vi "QueuedMessageHandler 1.vi"   [LabVIEW 2012]
doc: "Use this template to build a queued message handler design pattern.\nNote: This template does not contain the most recent programming guidelines recommended by National Instruments. For a complete, project-based implementation of the Queued Message Handler pattern, use the Create Project dialog box instead of this template."
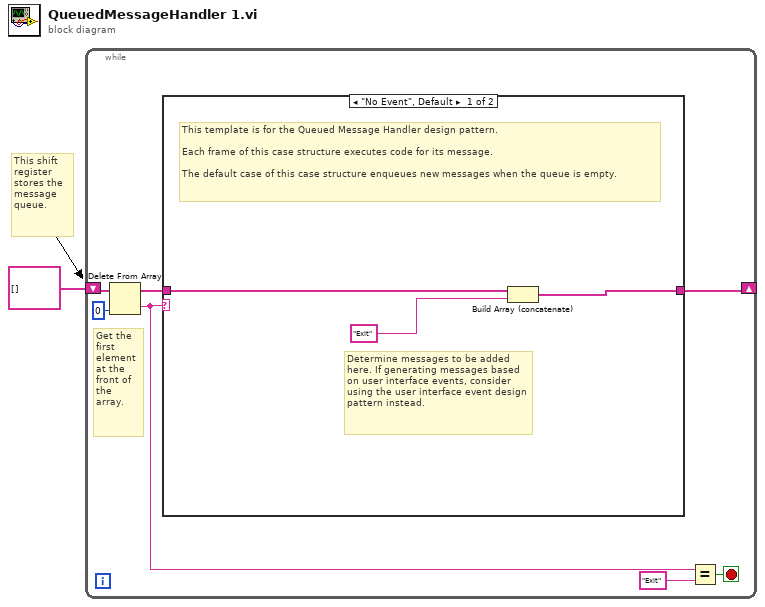
[diagram p0: block diagram]
diagram:
  # "This shift register stores the message queue."
  n1 = while {
    shift-right: [w4] -> _
    shift-left: string[] [] -> [w7]
    stop <- w8 stop-if-true
    # "Get the first element at the front of the array."
    n2 = Delete From Array(array=w7, index=0) -> (deleted portion=w6:string, array with subset deleted=w5:string[])  [unwired: 1 in]
    n3 = case shown="\"No Event\", Default" w6 {
      tunnel: w5 -> [w11 w12]
      tunnel: [w10 w12] -> w4
      frame "No Event", Default {
        # "Determine messages to be added here. If generating messages based on user interface events, consider using the user interface event design pattern instead."
        # "This template is for the Queued Message Handler design pattern.\n\nEach frame of this case structure executes code for its message.\n\nThe default case of this case structure enqueues new messages when the queue is empty."
        n4 = Build Array (concatenate)(w11, "Exit") -> (w10:string[])
      }
      frame "Exit" {
        # "Code in this case will execute once on exit."
      }
    }
    n5 = Equal?(x=w6, y="Exit") -> (x = y?=w8:bool)
  }
